vi "Init Condition.vi"(5 "Sequencing":refnum<class "MessageQ.lvclass">, 6 "Variables":refnum<class "Variables.lvclass">, 7 "VolatusAPI":refnum<class "VolatusAPI.lvclass">, 8 "error in (no error)":refnum<class "MultiErrors.lvclass">, 10 "Condition Config":refnum<class "Condition Config.lvclass">, 11 "HighLimit Condition in":refnum<class "HighLimit Condition.lvclass">) -> (0 "error out":refnum<class "MultiErrors.lvclass">, 3 "HighLimit Condition out":refnum<class "HighLimit Condition.lvclass">)   [LabVIEW 2020, in "VolatusSeq.lvlib" / "HighLimit Condition.lvclass"]
uses:
  HighLimit Condition.lvclass
  VolatusErrorUtilities/MultiErrors/MultiErrors.lvclass
  Volatus/VolatusAPI/VolatusAPI.lvclass
  VolatusSeqConfig/Condition Config/Condition Config.lvclass
  Volatus/MessageQ/MessageQ.lvclass
  VolatusSeqConfig/HighLimit Condition Config/HighLimit Condition Config.lvclass
  VolatusSeqConfig/HighLimit Condition Config/HighLimit Condition Config.lvclass/HighLimit Condition Config.ctl
  Volatus/VolatusAPI/VolatusAPI.lvclass/VolatusAPI.ctl
  HighLimit Condition.lvclass/HighLimit Condition.ctl
  lv-vecto/Vecto/ChannelService/Lookup Double Channel.vi
  Condition Value/Condition Value.lvclass
  Variables/Variables.lvclass
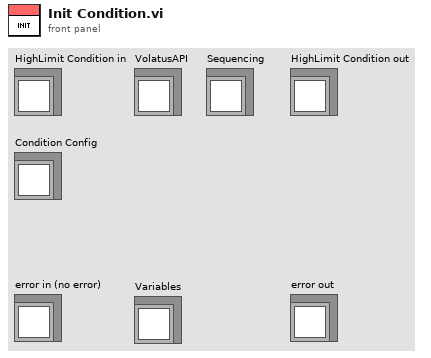
[diagram p1: front panel]
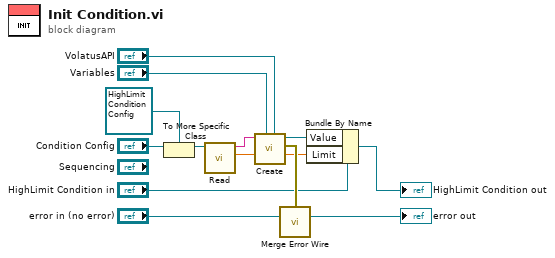
[diagram p0: block diagram]
diagram:
  n1 = To More Specific Class(target class=refnum<class "HighLimit Condition Config.lvclass"> refnum ("VolatusSeqConfig.lvlib:HighLimit Condition Config.lvclass"), reference="Condition Config") -> (specific class reference=w9:refnum<class "HighLimit Condition Config.lvclass">)  [unwired: 1 in, 1 out]
  n2 = call "Read.vi"("HighLimit Condition Config in"=w9) -> ("Limit"=w7:dbl, "Channel"=w3:string)  [unwired: 9 in]
  n3 = call "Create.vi"("VolatusAPI"="VolatusAPI", "Variables"="Variables", "Source Name"=w3) -> ("error out"=w13:errorcluster, "Condition Value out"=w4:refnum<class "Condition Value.lvclass">)  [unwired: 7 in]
  n4 = call "Merge Error Wire.vi"("error in (no error)"=w13, "MultiErrors in"="error in (no error)") -> ("MultiErrors out"=→"error out":refnum<class "MultiErrors.lvclass">)  [unwired: 13 in]
  n5 = Bundle By Name(cluster="HighLimit Condition in", "Value"=w4, "Limit"=w7) -> (→"HighLimit Condition out":refnum<class "HighLimit Condition.lvclass">)
